vi "Chroma 1905x Series VI Tree.vi"   [LabVIEW 2025]
doc: "Contact Chroma\nTEL: +886-2-2298-3855 \nTEL: +886-3-397-5788 \nFAX: +886-2-2298-3596\nFAX: +886-3-327-4703 \nURL: http://www.chromaate.com \nE-mail: chroma@chroma.com.tw"
uses:
  <instrlib>/Chroma 19052/Chroma 19052.lvlib
panel:
  # "See Block Diagram\nFor VI Tree"
  # "Chroma 1905x Series LabView Driver\nWebsite: www.chroma.com"
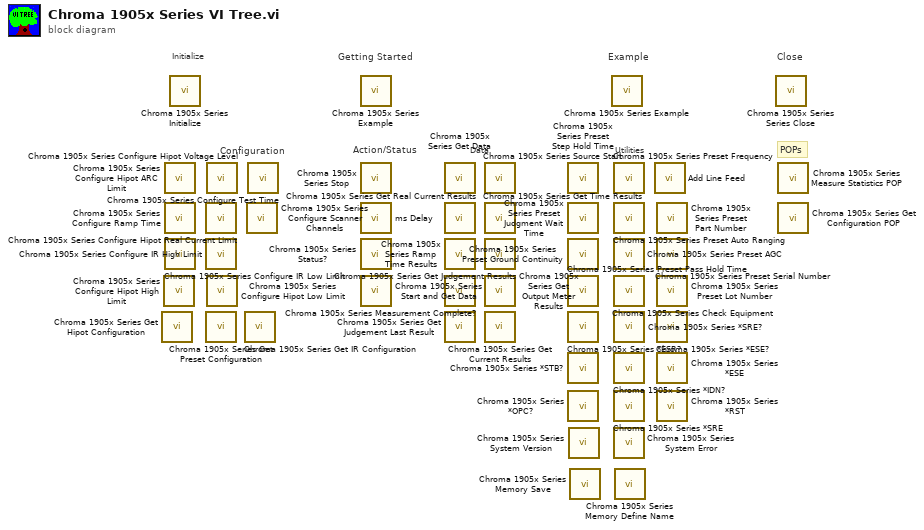
[diagram p0: block diagram]
diagram:
  # "POPs"
  # "Getting Started"
  # "Data"
  # "Example"
  # "Close"
  # "Utilities"
  # "Action/Status"
  # "Configuration"
  # "Initialize"
  n1 = call "Chroma 1905x Series Get Hipot Configuration.vi"() -> ()  [unwired: 8 in, 12 out]
  n2 = call "Chroma 1905x Series Configure Hipot High Limit.vi"() -> ()  [unwired: 5 in, 2 out]
  n3 = call "Chroma 1905x Series Configure Hipot ARC Limit.vi"() -> ()  [unwired: 5 in, 2 out]
  n4 = call "Chroma 1905x Series Configure Ramp Time.vi"() -> ()  [unwired: 5 in, 2 out]
  n5 = call "Chroma 1905x Series Configure IR Low Limit.vi"() -> ()  [unwired: 5 in, 2 out]
  n6 = call "Chroma 1905x Series Initialize.vi"() -> ()  [unwired: 4 in, 3 out]
  n7 = call "Chroma 1905x Series Configure Hipot Real Current Limit.vi"() -> ()  [unwired: 5 in, 2 out]
  n8 = call "Chroma 1905x Series Configure IR High Limit.vi"() -> ()  [unwired: 5 in, 2 out]
  n9 = call "Chroma 1905x Series Get Preset Configuration.vi"() -> ()  [unwired: 6 in, 14 out]
  n10 = call "Chroma 1905x Series Configure Hipot Voltage Level.vi"() -> ()  [unwired: 5 in, 2 out]
  n11 = call "Chroma 1905x Series Configure Hipot Low Limit.vi"() -> ()  [unwired: 5 in, 2 out]
  n12 = call "Chroma 1905x Series Get IR Configuration.vi"() -> ()  [unwired: 11 in, 9 out]
  n13 = call "Chroma 1905x Series Configure Scanner Channels.vi"() -> ()  [unwired: 5 in, 2 out]
  n14 = call "Chroma 1905x Series Configure Test Time.vi"() -> ()  [unwired: 5 in, 2 out]
  n15 = call "Chroma 1905x Series Example.vi"() -> ()  [unwired: 1 in]
  n16 = call "Chroma 1905x Series Stop.vi"() -> ()  [unwired: 3 in, 2 out]
  n17 = call <instrlib>:"ms Delay.vi"() -> ()  [unwired: 3 in, 2 out]
  n18 = call "Chroma 1905x Series Status?.vi"() -> ()  [unwired: 3 in, 3 out]
  n19 = call "Chroma 1905x Series Start and Get Data.vi"() -> ()  [unwired: 4 in, 6 out]
  n20 = call "Chroma 1905x Series Get Data.vi"() -> ()  [unwired: 7 in, 3 out]
  n21 = call "Chroma 1905x Series Get Real Current Results.vi"() -> ()  [unwired: 3 in, 3 out]
  n22 = call "Chroma 1905x Series Ramp Time Results.vi"() -> ()  [unwired: 3 in, 3 out]
  n23 = call "Chroma 1905x Series Measurement Complete?.vi"() -> ()  [unwired: 3 in, 3 out]
  n24 = call "Chroma 1905x Series Get Judgement Last Result.vi"() -> ()  [unwired: 3 in, 3 out]
  n25 = call "Chroma 1905x Series Source Start.vi"() -> ()  [unwired: 8 in, 2 out]
  n26 = call "Chroma 1905x Series Get Time Results.vi"() -> ()  [unwired: 3 in, 3 out]
  n27 = call "Chroma 1905x Series Get Judgement Results.vi"() -> ()  [unwired: 3 in, 3 out]
  n28 = call "Chroma 1905x Series Get Output Meter Results.vi"() -> ()  [unwired: 3 in, 3 out]
  n29 = call "Chroma 1905x Series Get Current Results.vi"() -> ()  [unwired: 3 in, 3 out]
  n30 = call "Chroma 1905x Series Preset Step Hold Time.vi"() -> ()  [unwired: 3 in, 2 out]
  n31 = call "Chroma 1905x Series Preset Judgment Wait Time.vi"() -> ()  [unwired: 3 in, 2 out]
  n32 = call "Chroma 1905x Series Preset Ground Continuity.vi"() -> ()  [unwired: 3 in, 2 out]
  n33 = call "Chroma 1905x Series Preset Pass Hold Time.vi"() -> ()  [unwired: 3 in, 2 out]
  n34 = call "Chroma 1905x Series *ESR?.vi"() -> ()  [unwired: 3 in, 3 out]
  n35 = call "Chroma 1905x Series *STB?.vi"() -> ()  [unwired: 3 in, 3 out]
  n36 = call "Chroma 1905x Series *OPC?.vi"() -> ()  [unwired: 4 in, 2 out]
  n37 = call "Chroma 1905x Series System Version.vi"() -> ()  [unwired: 3 in, 3 out]
  n38 = call "Chroma 1905x Series Memory Save.vi"() -> ()  [unwired: 4 in, 2 out]
  n39 = call "Chroma 1905x Series Example.vi"() -> ()  [unwired: 1 in]
  n40 = call "Chroma 1905x Series Preset Frequency.vi"() -> ()  [unwired: 3 in, 2 out]
  n41 = call "Chroma 1905x Series Preset Auto Ranging.vi"() -> ()  [unwired: 3 in, 2 out]
  n42 = call "Chroma 1905x Series Preset AGC.vi"() -> ()  [unwired: 3 in, 2 out]
  n43 = call "Chroma 1905x Series Check Equipment.vi"() -> ()  [unwired: 7 in, 3 out]
  n44 = call "Chroma 1905x Series *SRE?.vi"() -> ()  [unwired: 3 in, 3 out]
  n45 = call "Chroma 1905x Series *IDN?.vi"() -> ()  [unwired: 3 in, 3 out]
  n46 = call "Chroma 1905x Series *SRE.vi"() -> ()  [unwired: 4 in, 2 out]
  n47 = call "Chroma 1905x Series System Error.vi"() -> ()  [unwired: 3 in, 3 out]
  n48 = call "Chroma 1905x Series Memory Define Name.vi"() -> ()  [unwired: 4 in, 2 out]
  n49 = call <instrlib>:"Add Line Feed.vi"() -> ()  [unwired: 1 in, 1 out]
  n50 = call "Chroma 1905x Series Preset Part Number.vi"() -> ()  [unwired: 3 in, 2 out]
  n51 = call "Chroma 1905x Series Preset Serial Number.vi"() -> ()  [unwired: 3 in, 2 out]
  n52 = call "Chroma 1905x Series Preset Lot Number.vi"() -> ()  [unwired: 3 in, 2 out]
  n53 = call "Chroma 1905x Series *ESE?.vi"() -> ()  [unwired: 3 in, 3 out]
  n54 = call "Chroma 1905x Series *ESE.vi"() -> ()  [unwired: 4 in, 2 out]
  n55 = call "Chroma 1905x Series *RST.vi"() -> ()  [unwired: 4 in, 2 out]
  n56 = call "Chroma 1905x Series Series Close.VI"() -> ()  [unwired: 4 in, 1 out]
  n57 = call "Chroma 1905x Series Measure Statistics POP.vi"() -> ()  [unwired: 4 in, 5 out]
  n58 = call "Chroma 1905x Series Get Configuration POP.vi"() -> ()  [unwired: 7 in, 2 out]
